vi "simpleAccRead.vi"() -> ()   [LabVIEW 2019]
uses:
  <vilib>/myRIO/Instrument Drivers/Onboard IO/I2C/typedefs/I2C Transfer Rate.ctl
  <vilib>/myRIO/Instrument Drivers/Onboard IO/I2C/I2C.lvlib
  <vilib>/myRIO/Instrument Drivers/Onboard IO/I2C/typedefs/I2C Configuration.ctl
  <vilib>/myRIO/Common/Instrument Driver Framework/myRIO v1.0/I2C/typedefs/I2C Channels Enum.ctl
  <vilib>/myRIO/Common/Instrument Driver Framework/Utilities/typedefs/Generic FPGA Reference.ctl
  <vilib>/myRIO/Common/Instrument Driver Framework/Utilities/typedefs/myRIO v1.0 Reference.ctl
  <vilib>/myRIO/Common/Instrument Driver Framework/Utilities/typedefs/Hardware Version Enum.ctl
  <vilib>/myRIO/Common/Instrument Driver Framework/Utilities/typedefs/myRIO Generic Hardware Reference.ctl
  <vilib>/myRIO/Instrument Drivers/Onboard IO/I2C/typedefs/I2C Reference.ctl
  <vilib>/userdefined/High Color/nirio_resource_hc.ctl
  <vilib>/myRIO/Common/Instrument Driver Framework/myRIO v1.0/I2C/vis/myRIO v1.1 Open I2C.vi
  <vilib>/myRIO/Instrument Drivers/Onboard IO/I2C/vis/myRIO I2C Open.xnode
  <vilib>/myRIO/Instrument Drivers/Onboard IO/I2C/typedefs/I2C User Configuration.ctl
  <vilib>/myRIO/Instrument Drivers/Utilities/Utilities.lvlib
  <vilib>/platform/TimedLoop/XDataNode/XDataNode.xnode
  <vilib>/Platform/TimedLoop/XDataNode/nitl_modes.ctl
  <vilib>/Platform/TimedLoop/XDataNode/XDNodeRunTimeDep.lvlib
  <vilib>/Platform/TimedLoop/XDataNode/wakeup.ctl
  <vilib>/Platform/TimedLoop/XDataNode/timing_clust.ctl
  <vilib>/ptbypt/NI_PtbyPt.lvlib
panel:
  out "czas":u32
  in  "Period":i64=5
  out "Histogram Graph":T1(graph)
  out "x != 0?":bool
  out "byte count":u32
  out "Waveform Graph":waveform(dbl)[](graph)
  in  "stop":bool
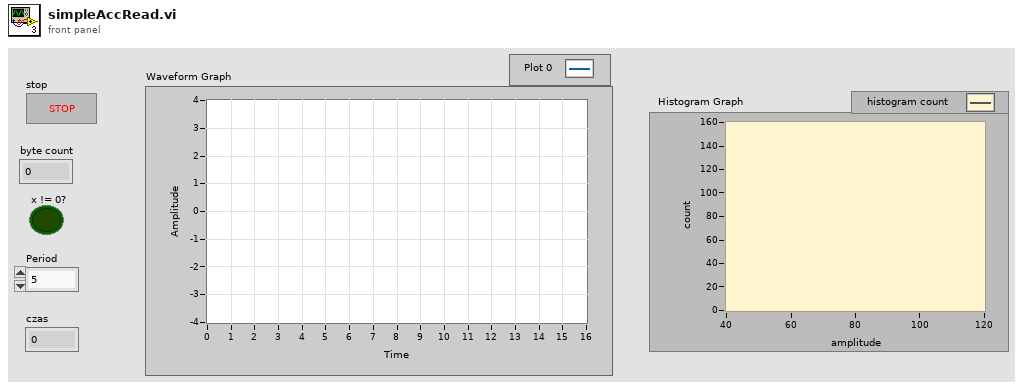
[diagram p1: front panel]
types:
  T1 = cluster{"X Values":dbl[], "Histogram: h(x)":i32[]}
  T2 = typedef "I2C.lvlib/I2C User Configuration.ctl" = cluster{"I2C Transfer Rate":T3}
  T3 = typedef "I2C.lvlib/I2C Transfer Rate.ctl" = enum16{"Standard mode (100 kbps)", "Fast mode (400 kbps)"}
  T4 = typedef "I2C.lvlib/I2C Reference.ctl" = cluster{"myRIO Reference":T5, "I2C Channels Enum":T9, "I2C Configuration":T10}
  T5 = typedef "myRIO Generic Hardware Reference.ctl" = cluster{"myRIO Model":T6, "myRIO Hardware Reference":T7}
  T6 = typedef "Hardware Version Enum.ctl" = enum16{"Unknown", "myRIO-1900", "myRIO-1950", "roboRIO", "NI ELVIS RIO CM", "ELVIS III"}
  T7 = typedef "myRIO v1.0 Reference.ctl" = cluster{"Generic FPGA Reference":T8, "Allow multiple opens":bool}
  T8 = typedef "Generic FPGA Reference.ctl" = refnum<k20>
  T9 = typedef "I2C Channels Enum.ctl" = enum16{"Not Connected", "A/I2C", "B/I2C", "I2C/I2C"}
  T10 = typedef "I2C.lvlib/I2C Configuration.ctl" = cluster{"I2C Transfer Rate":T3}
  T11 = typedef "XDNodeRunTimeDep.lvlib/timing_clust.ctl" = cluster{"Expected End [f-1]":u64, "Actual End [f-1]":u64, "Finished Late? [f-1]":bool, "Expected End [i-1]":u64, "Actual End [i-1]":u64, "Finished Late? [i-1]":bool, "Expected Start [i]":u64, "Actual Start [i]":u64, "Expected Start [f]":u64, "Actual Start [f]":u64, "Source Name":string, "Structure Name":string, "Period":i64, "Deadline":i64, "Offset":i64, "Start":i64, "Priority":i32, "Timeout":i32, "Mode":T12, "Wakeup Reason":T13, "Error":errorcluster, "Source Type":string, "Secondary Source Type":string, "Global End Time":u64, "Global Start Time":u64, "Frame Duration":u64, "Iteration Duration":u64, "Assigned CPU":i32, "I/O Scan Engine Mode":u32}
  T12 = typedef "XDNodeRunTimeDep.lvlib/nitl_modes.ctl" = enum32{"No Change", "Process missed periods, maintain original phase", "Discard missed periods, maintain original phase", "Process missed periods, ignore original phase", "Discard missed periods, ignore original phase"}
  T13 = typedef "XDNodeRunTimeDep.lvlib/wakeup.ctl" = enum32{"Normal", "Aborted", "Asynchronous wakeup", "Timing source error", "Timed loop error", "Timeout"}
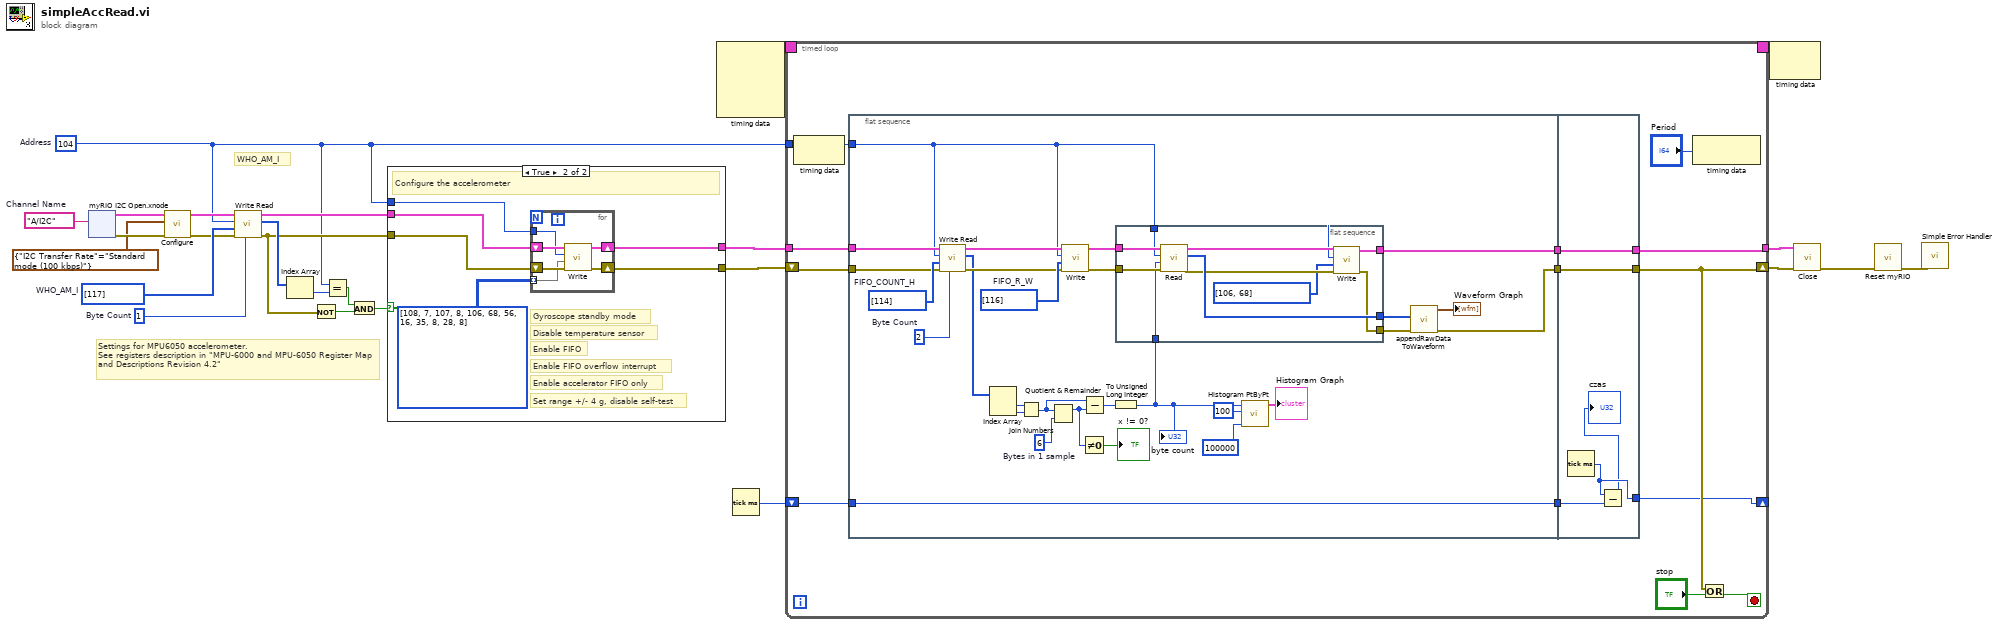
[diagram p0: block diagram]
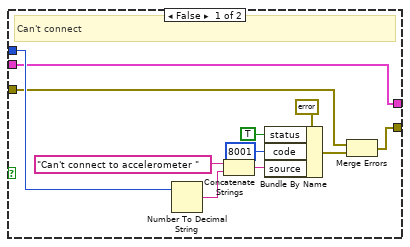
[diagram p2: hidden frame]
diagram:
  w8 = u8 104  # Address
  w21 = u32 1  # Byte Count
  w20 = u8[] [117]  # WHO_AM_I
  w24 = tag "A/I2C"  # Channel Name
  # "Settings for MPU6050 accelerometer.\nSee registers description in \"MPU-6000 and MPU-6050 Register Map and Descriptions Revision 4.2\""
  # "WHO_AM_I"
  n1 = xnode ("myRIO I2C Open.xnode")("Channel Name"=w24) -> ("error out"=w25:errorcluster, "I2C Ref Out"=w12:T4)  [unwired: 2 in]
  n2 = call <vilib>:"Configure.vi"("error in (no error)"=w25, "I2C User Configuration"=T2 {"I2C Transfer Rate"=enum."Standard mode (100 kbps)"}, "I2C Ref In"=w12) -> ("error out"=w14:errorcluster, "I2C Ref Out"=w15:T4)  [unwired: 7 in]
  n3 = call <vilib>:"Write Read.vi"("Byte Count"=w21, "error in (no error)"=w14, "Bytes to Write"=w20, "Slave Address (7-bit)"=w8, "I2C Ref In"=w15) -> ("error out"=w17:errorcluster, "Bytes Read"=w22:u8[], "I2C Ref Out"=w19:T4)  [unwired: 3 in]
  n4 = Index Array(array=w22) -> (element=w23:u8)  [unwired: 1 in]
  n5 = Not(x=w17) -> (.not. x?=w16:bool)
  n6 = Equal?(x=w8, y=w23) -> (x = y?=w18:bool)
  n7 = And(x=w18, y=w16) -> (x .and. y?=w13:bool)
  n8 = case shown="True" w13 {
    tunnel: w8 -> [w34 w39]
    tunnel: w19 -> [w26 w42]
    tunnel: w17 -> [w29 w41]
    tunnel: [w27 w38] -> w10
    tunnel: [w26 w37] -> w9
    frame False {
      # "Can't connect"
      n9 = Number To Decimal String(number=w34) -> (decimal integer string=w31:string)  [unwired: 1 in]
      n10 = Concatenate Strings("Can't connect to accelerometer " ("source"), w31) -> (w33:string)
      n11 = Bundle By Name(cluster=errorcluster {"status"=FALSE, "code"=0, "source"=""} ("error constant"), "status"=TRUE, "code"=8001, "source"=w33) -> (w28:errorcluster)
      n12 = Merge Errors(w29, w28) -> (w27:errorcluster)
    }
    frame True {
      # "Enable accelerator FIFO only"
      # "Disable temperature sensor"
      # "Gyroscope standby mode"
      # "Set range +/- 4 g, disable self-test"
      # "Enable FIFO"
      # "Enable FIFO overflow interrupt"
      # "Configure the accelerometer"
      n13 = for {
        shift-right: [w45] -> w38
        shift-left: w41 -> [w48]
        shift-right: [w46] -> w37
        shift-left: w42 -> [w47]
        tunnel: u8[][] [[108, 7], [107, 8], [106, 68], [56, 16], [35, 8], [28, 8]] ("Bytes to Write") -> [w44] mode=indexing
        tunnel: w39 -> [w43]
        n14 = call <vilib>:"Write.vi"("error in (no error)"=w48, "Bytes to Write"=w44, "Slave Address (7-bit)"=w43, "I2C Ref In"=w47) -> ("error out"=w45:errorcluster, "I2C Ref Out"=w46:T4)  [unwired: 6 in]
      }
    }
  }
  n15 = node-c288() -> (w3:T11)  [unwired: 4 in]
  n16 = Tick Count (ms)() -> (millisecond timer value=w1:u32)
  n17 = timed-loop {
    tunnel: w9 -> [w60]
    tunnel: w8 -> [w55]
    shift-right: [w57] -> w5
    shift-left: w10 -> [w59]
    tunnel: [w56] -> w6
    timing: w3 -> [_]
    timing-out: [_] -> w2
    shift-right: [w49] -> _
    shift-left: w1 -> [w51]
    stop <- w58 stop-if-true
    n18 = node-c288() -> ()  [unwired: 1 in, 1 out]
    n19 = flat-sequence {
      tunnel: w60 -> [w84]
      tunnel: w59 -> [w83]
      tunnel: w55 -> [w63]
      tunnel: [w74] -> w53
      tunnel: [w64] -> w52
      tunnel: w51 -> [w62]
      tunnel: [w62] -> w50
      tunnel: [w103] -> w56
      tunnel: [w104] -> w57
      tunnel: w53 -> [w104]
      tunnel: w52 -> [w103]
      tunnel: w50 -> [w102]
      tunnel: [w101] -> w49
      frame #0 {
        w73 = u16 6  # Bytes in 1 sample
        w85 = u8[] [114]  # FIFO_COUNT_H
        w86 = u32 2  # Byte Count
        w89 = u8[] [116]  # FIFO_R_W
        n20 = call <vilib>:"Write Read.vi"("Byte Count"=w86, "error in (no error)"=w83, "Bytes to Write"=w85, "Slave Address (7-bit)"=w63, "I2C Ref In"=w84) -> ("error out"=w82:errorcluster, "Bytes Read"=w77:u8[], "I2C Ref Out"=w81:T4)  [unwired: 3 in]
        n21 = Index Array(array=w77) -> (element #1=w80:u8, element #2=w78:u8)  [unwired: 2 in]
        n22 = Join Numbers(hi=w80, lo=w78) -> ((hi.lo)=w79:u16)
        n23 = Quotient & Remainder(x=w79, y=w73) -> (x-y*floor(x/y)=w71:u16)  [unwired: 1 out]
        n24 = call <vilib>:"Write.vi"("error in (no error)"=w82, "Bytes to Write"=w89, "Slave Address (7-bit)"=w63, "I2C Ref In"=w81) -> ("error out"=w87:errorcluster, "I2C Ref Out"=w88:T4)  [unwired: 6 in]
        n25 = Not Equal To 0?(x=w71) -> (x != 0?=→"x != 0?":bool)
        n26 = Subtract(x=w79, y=w71) -> (x-y=w76:u16)
        n27 = To Unsigned Long Integer(number=w76) -> (unsigned 32bit integer=w69:u32)
        "byte count" <- w69
        n28 = flat-sequence {
          tunnel: w88 -> [w99]
          tunnel: w87 -> [w98]
          tunnel: [w97] -> w72
          tunnel: w69 -> [w96]
          tunnel: [w93] -> w65
          tunnel: [w92] -> w64
          tunnel: w63 -> [w90]
          frame #0 {
            n29 = call <vilib>:"Read.vi"("error in (no error)"=w98, "Byte Count"=w96, "Slave Address (7-bit)"=w90, "I2C Ref In"=w99) -> ("error out"=w94:errorcluster, "Bytes Read"=w97:u8[], "I2C Ref Out"=w95:T4)  [unwired: 4 in]
            n30 = call <vilib>:"Write.vi"("error in (no error)"=w94, "Bytes to Write"=u8[] [106, 68], "Slave Address (7-bit)"=w90, "I2C Ref In"=w95) -> ("error out"=w93:errorcluster, "I2C Ref Out"=w92:T4)  [unwired: 6 in]
          }
        }
        n31 = call <vilib>:"Histogram PtByPt.vi"("sample length"=100000, "intervals"=100, "x"=w69) -> ("Histogram Graph"=→"Histogram Graph":T1)  [unwired: 5 in, 3 out]
        n32 = call "appendRawDataToWaveform.vi"("ErrorIn"=w65, "AccelerationRawData"=w72) -> ("ErrorOut"=w74:errorcluster, "AccelerationDataOut"=→"Waveform Graph":waveform(dbl)[])  [unwired: 7 in, 1 out]
      }
      frame #1 {
        n33 = Tick Count (ms)() -> (millisecond timer value=w101:u32)
        n34 = Subtract(x=w101, y=w102) -> (x-y=→"czas":u32)
      }
    }
    n35 = node-c288("Period") -> ()  [unwired: 1 out]
    n36 = Or(x=w57, y="stop") -> (x .or. y?=w58:bool)
  }
  n37 = node-c288(w2) -> ()  [unwired: 1 out]
  n38 = call <vilib>:"Close.vi"("error in (no error)"=w5, "I2C Ref In"=w6) -> ("error out"=w7:errorcluster)  [unwired: 9 in]
  n39 = call <vilib>:"Reset myRIO.vi"("error in (no error)"=w7) -> ("error out"=w4:errorcluster)  [unwired: 10 in]
  n40 = call <vilib>:"Simple Error Handler.vi"("error in (no error)"=w4) -> ()  [unwired: 4 in, 5 out]
